vi "Read Position.vi"(8 "error in (no error)":errorcluster, 11 "BC_Evolut_1D.lvclass in":refnum<class "NI_BC_Evolut_1D.lvclass">) -> (0 "error out":errorcluster, 2 "BC position 1D":T1 items=["Start X", "End X"], 3 "BC_Evolut_1D.lvclass out":refnum<class "NI_BC_Evolut_1D.lvclass">)   [LabVIEW 2020, in "NI_PDE.lvlib" / "NI_BC_Evolut_1D.lvclass"]
uses:
  <vilib>/gmath/pde.llb/BCClass/BC_Evolut_1D/NI_BC_Evolut_1D.lvclass
  <vilib>/gmath/pde.llb/Common/PDE_BC Position 1D.ctl
  <vilib>/gmath/pde.llb/BCClass/BC_Evolut_1D/NI_BC_Evolut_1D.lvclass/NI_BC_Evolut_1D.ctl
  <vilib>/gmath/NI_PDE.lvlib
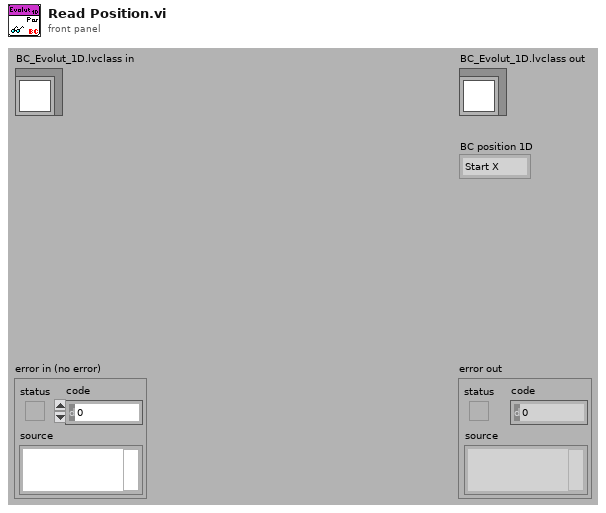
[diagram p1: front panel]
types:
  T1 = typedef "NI_PDE.lvlib/PDE_BC Position 1D.ctl" = i32
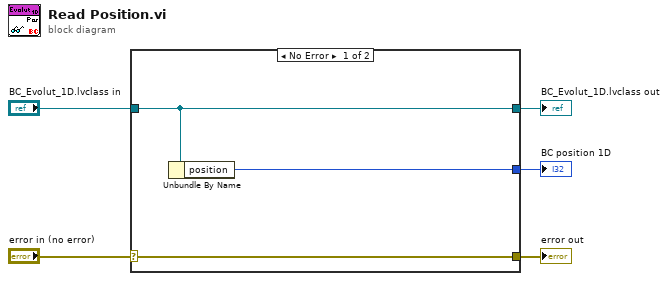
[diagram p0: block diagram]
diagram:
  n1 = case shown="No Error" "error in (no error)" {
    selector: "error in (no error)" -> [w8 w9]
    tunnel: [w8 w9] -> w4
    tunnel: [w7 w10] -> w2
    tunnel: "BC_Evolut_1D.lvclass in" -> [w7 w10]
    tunnel: [w6 _] -> w1
    frame No Error {
      n2 = Unbundle By Name(w7) -> ("position"=w6:T1)
    }
    frame Error {
    }
  }
  "error out" <- w4
  "BC_Evolut_1D.lvclass out" <- w2
  "BC position 1D" <- w1
